vi "ATMonochromator_getNextSample_timestamp.vi"(8 "error in (no error)":errorcluster, 11 "timestamp_Ctl":T1) -> (0 "error out":errorcluster, 2 "function return":i32, 3 "timestamp_Ctl out":T1)   [LabVIEW 2016, in "SALLV_ATMonochromator.lvlib"]
doc: "int ATMonochromator_shm_getNextSample_timestampLV(ATMonochromator_timestampLV *timestamp_Ctl );"
uses:
  SALLV_ATMonochromator.lvlib
  DataTypes/timestamp.ctl
  SALLV_ATMonochromator.so
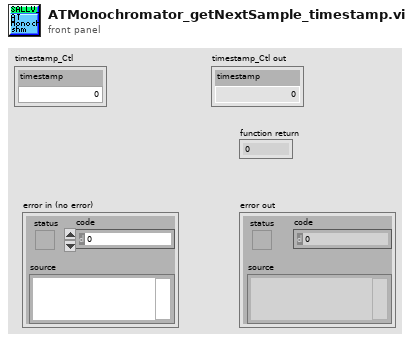
[diagram p1: front panel]
types:
  T1 = typedef "SALLV_ATMonochromator.lvlib/timestamp.ctl" = cluster{"timestamp":dbl}
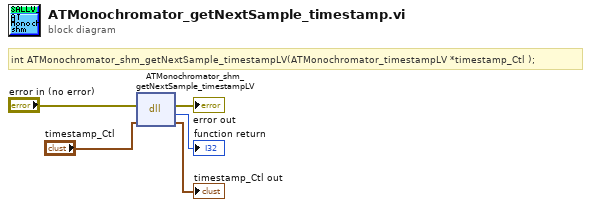
[diagram p0: block diagram]
diagram:
  # "int ATMonochromator_shm_getNextSample_timestampLV(ATMonochromator_timestampLV *timestamp_Ctl );"
  n1 = dll-call lib="home/harini/tcs/SALLV_ATMonochromator/SALLV_ATMonochromator.*" fn="ATMonochromator_shm_getNextSample_timestampLV"(error in="error in (no error)", "timestamp_Ctl"="timestamp_Ctl") -> (error out=→"error out":errorcluster, →"function return":i32, "timestamp_Ctl"=→"timestamp_Ctl out":T1)  [unwired: 2 in, 1 out]
